vi "York DIHB - Data Processing - Apply Calibration.vi"() -> ()   [LabVIEW 2020]
doc: "Load a datafile and calibration file. Apply the calibration to the data set, to convert from voltage to lbs force."
uses:
  Typedefs/Calibration Method - Enum.ctl
  <vilib>/Utility/file.llb/Read Delimited Spreadsheet (DBL).vi
panel:
  in  "Calibration Type":T1
  in  "Data File Path (TSV, CSV)":path
  out "First Pulse Data":waveform(dbl)(graph)
  in  "Calibration File (TSV)":path
  out "Calibrated Data":waveform(dbl)(graph)
  out "Samples":i32
  out "Sampling Rate (MHz)":dbl
  out "Sampling Period (s)":dbl
  out "Raw Data - Strain Amplifier Output (Volts)":waveform(dbl)(graph)
  out "Projectile Velocity (m/s)":dbl
  out "Strain Amplifier (Volts)":dbl[](array[numeric])
  out "Time (Seconds)":dbl[](array[numeric])
  # "Select data files and calibration type"
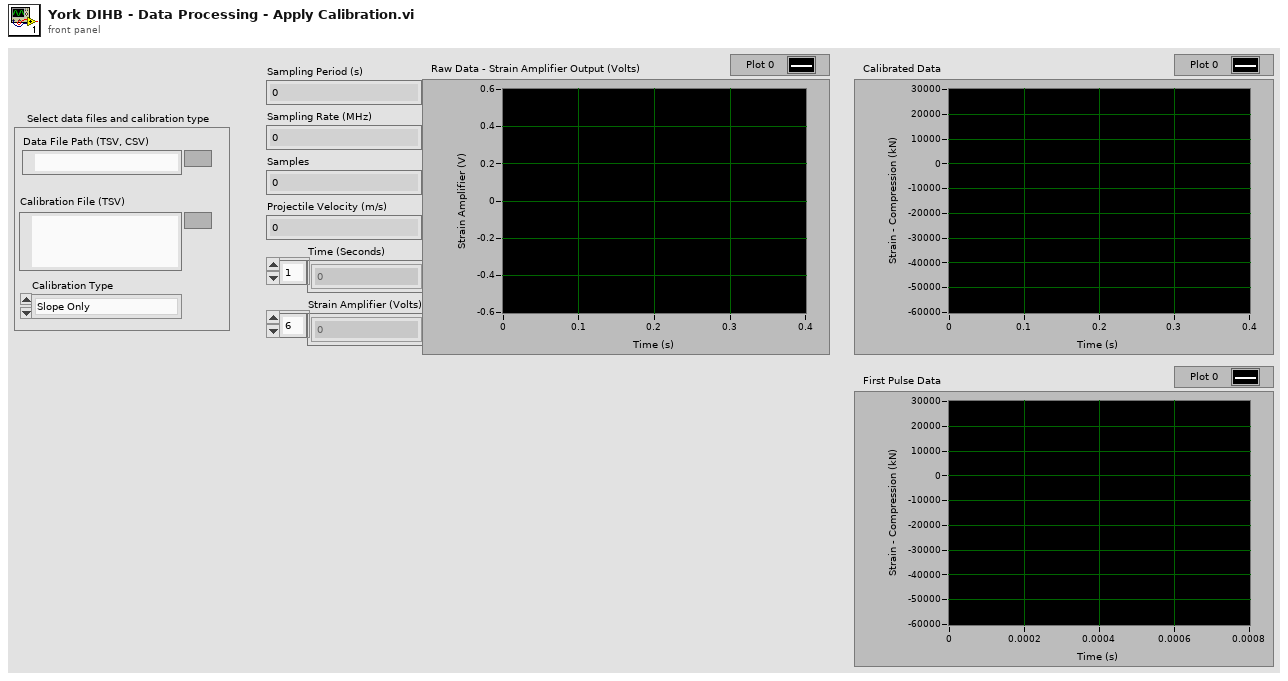
[diagram p1: front panel]
types:
  T1 = typedef "Calibration Method - Enum.ctl" = enum16{"Slope Only", "Slope and Offset"}
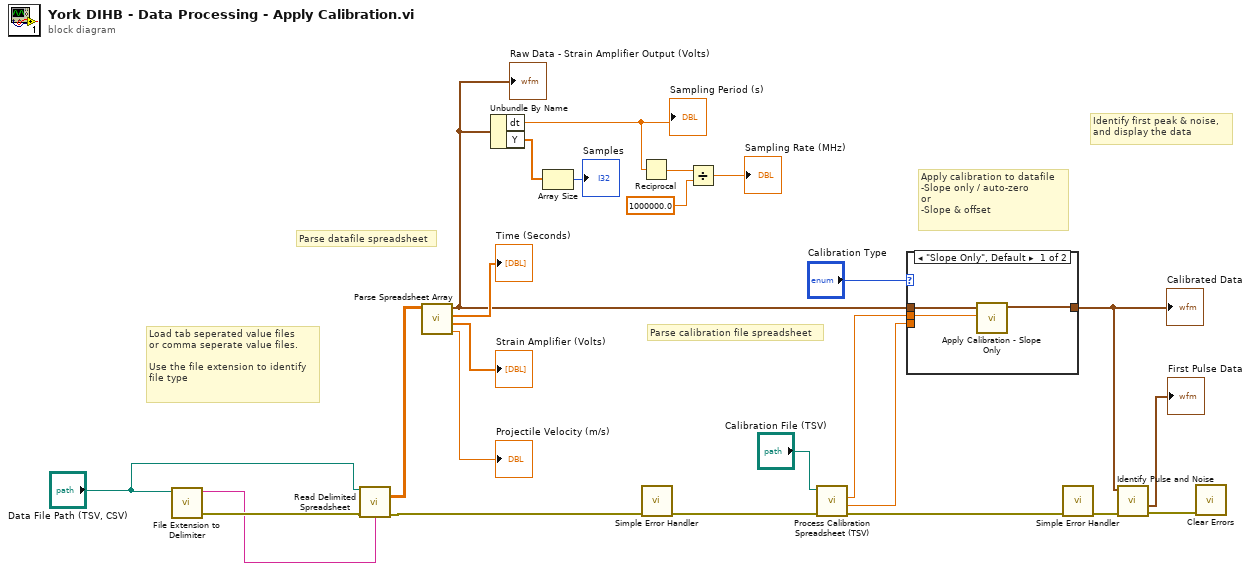
[diagram p0: block diagram]
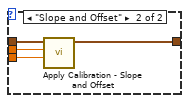
[diagram p2: hidden frame]
diagram:
  # "Identify first peak & noise,\nand display the data"
  # "Apply calibration to datafile\n-Slope only / auto-zero\nor\n-Slope & offset"
  # "Parse calibration file spreadsheet"
  # "Parse datafile spreadsheet"
  # "Load tab seperated value files \nor comma seperate value files.\n\nUse the file extension to identify\nfile type"
  n1 = call "File Extension to Delimiter.vi"("Data File Path"="Data File Path (TSV, CSV)") -> ("error out"=w13:errorcluster, "Delimiter"=w12:string)  [unwired: 9 in]
  n2 = call-poly <vilib>:"Read Delimited Spreadsheet.vi"("file path (dialog if empty)"="Data File Path (TSV, CSV)", "error in (no error)"=w13, "delimiter (\\t)"=w12) -> ("all rows"=w25:dbl[][], "error out"=w10:errorcluster)  [unwired: 7 in, 4 out]
  n3 = call "Parse Spreadsheet Array.vi"("all rows"=w25) -> ("Projectile Velocity (m/s)"=→"Projectile Velocity (m/s)":dbl, "Strain Amplifier (Volts)"=→"Strain Amplifier (Volts)":dbl[], "Time (Seconds)"=→"Time (Seconds)":dbl[], "Waveform"=w3:waveform(dbl))  [unwired: 7 in]
  "Raw Data - Strain Amplifier Output (Volts)" <- w3
  n4 = Unbundle By Name(w3) -> ("dt"=w21:dbl, "Y"=w16:dbl[])
  "Sampling Period (s)" <- w21
  n5 = Array Size(array=w16) -> (size(s)=→"Samples":i32)
  n6 = Reciprocal(x=w21) -> (1/x=w20:dbl)
  n7 = call <vilib>:"Simple Error Handler.vi"("error in (no error)"=w10) -> ("error out"=w9:errorcluster)  [unwired: 4 in, 4 out]
  n8 = Divide(x=w20, y=1000000.0) -> (x/y=→"Sampling Rate (MHz)":dbl)
  n9 = call "Process Calibration Spreadsheet (TSV).vi"("error in"=w9, "Calibration File"="Calibration File (TSV)") -> ("error out"=w7:errorcluster, "intercept"=w14:dbl, "slope"=w2:dbl)  [unwired: 5 in, 2 out]
  n10 = case shown="\"Slope Only\", Default" "Calibration Type" {
    tunnel: w14 -> [_ w32]
    tunnel: [w27 w31] -> w6
    tunnel: w3 -> [w28 w30]
    tunnel: w2 -> [w26 w29]
    frame "Slope Only", Default {
      n11 = call "Apply Calibration - Slope Only.vi"("slope"=w26, "Waveform in"=w28) -> ("Waveform out"=w27:waveform(dbl))  [unwired: 9 in]
    }
    frame "Slope and Offset" {
      n12 = call "Apply Calibration - Slope and Offset.vi"("intercept"=w32, "slope"=w29, "Waveform in"=w30) -> ("Waveform out"=w31:waveform(dbl))  [unwired: 8 in]
    }
  }
  "Calibrated Data" <- w6
  n13 = call <vilib>:"Simple Error Handler.vi"("error in (no error)"=w7) -> ("error out"=w8:errorcluster)  [unwired: 4 in, 4 out]
  n14 = call "Identify Pulse and Noise.vi"("error in"=w8, "Waveform In"=w6) -> ("error out"=w5:errorcluster, "Signal Waveform Out"=→"First Pulse Data":waveform(dbl))  [unwired: 5 in, 3 out]
  n15 = call <vilib>:"Clear Errors.vi"("error in (no error)"=w5) -> ()  [unwired: 5 in, 2 out]
